vi "Initialize (Test).vi"() -> ()   [LabVIEW 2025]
uses:
  <vilib>/Instr/_visa.llb/VISA Open Access Mode.ctl
  <instrlib>/SMS LabVIEW Drivers/Labview Drivers/Cryogenic Ltd SMSXXX.lvlib
  <vilib>/regexp/Match Regular Expression.xnode
panel:
  in  "EOT Character (auto)":string="auto"
  in  "Serial Configuration":T1={"Baud Rate"=9600, "Parity"=0, "Data Bits"=8, "Stop Bits"=10, "Flow Control"=0} {"Flow Control" items=["None", "XON/XOFF", "RTS/CTS", "XON/XOFF & RTS/CTS", "DTR/DSR", "XON/XOFF & DTR/DSR"]; "Stop Bits" items=["1.0"=10, "1.5"=15, "2.0"=20]; "Data Bits" items=["7"=7, "8"=8]; "Parity" items=["None", "Odd", "Even", "Mark", "Space"]; "Baud Rate" items=["300"=300, "600"=600, "1200"=1200, "2400"=2400, "4800"=4800, "9600"=9600, "19200"=19200]}
  out "error out":errorcluster
  out "VISA Resource Name Out":refnum<visa-resource-name>
  in  "ID Query (True)":bool=TRUE
  in  "error in":errorcluster
  in  "APS VISA  IN":refnum<visa-resource-name>
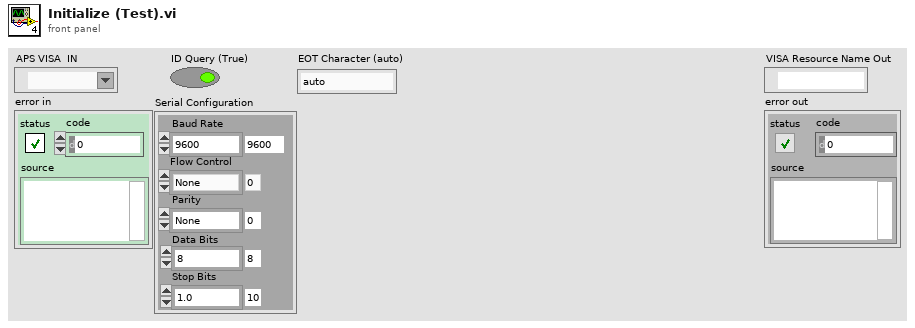
[diagram p1: front panel]
types:
  T1 = cluster{"Baud Rate":u32, "Parity":u16, "Data Bits":u16, "Stop Bits":u16, "Flow Control":u16}
  T2 = typedef "VISA Open Access Mode.ctl" = u32
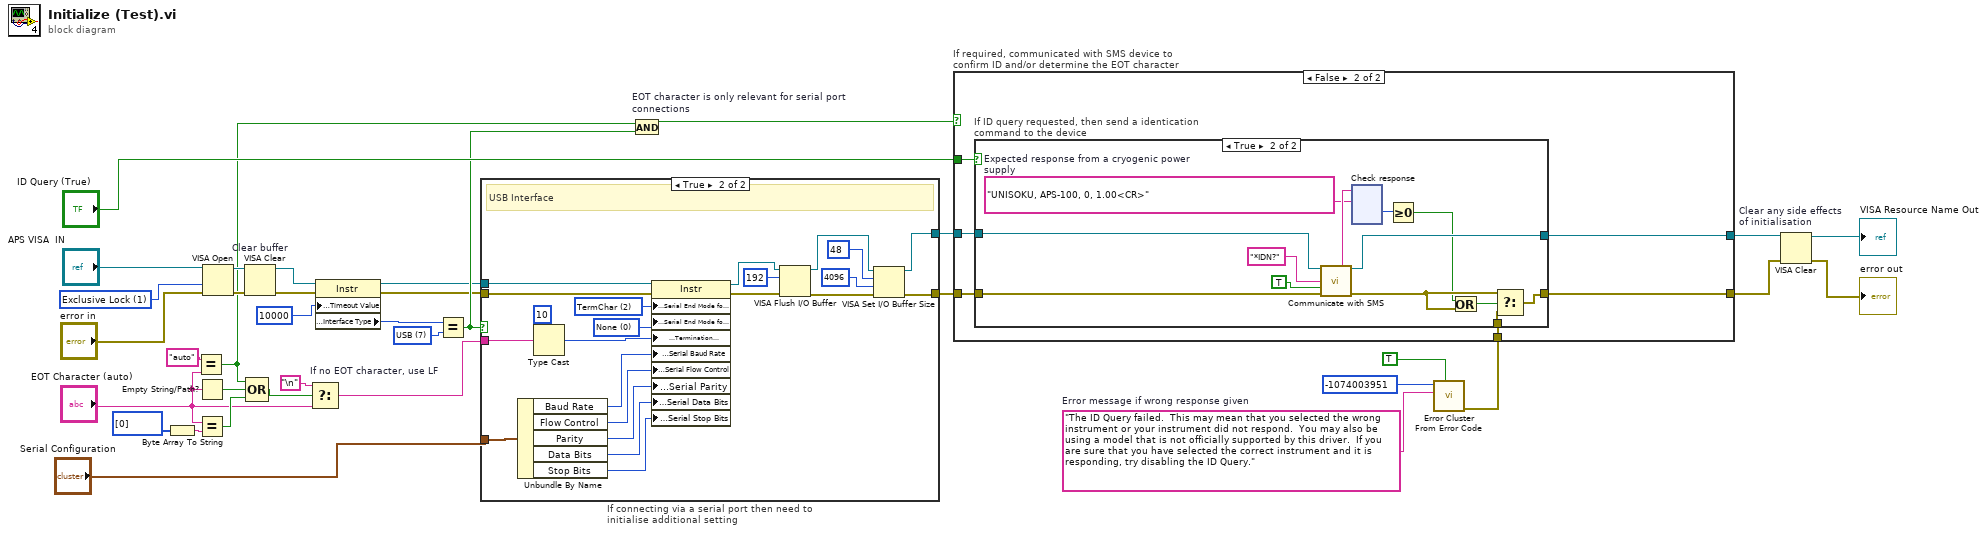
[diagram p0: block diagram]
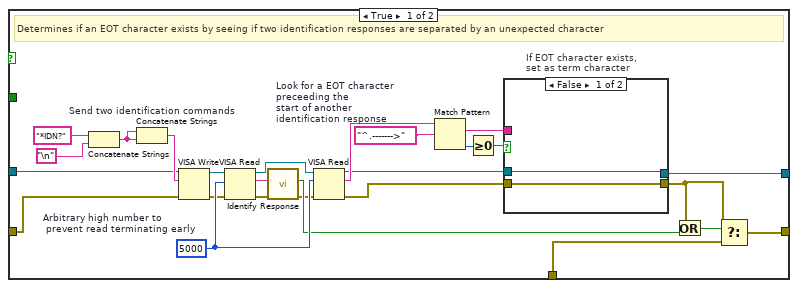
[diagram p2: hidden frame]
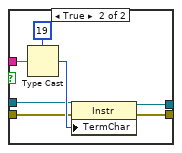
[diagram p3: hidden frame]
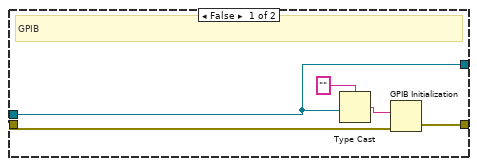
[diagram p5: hidden frame]
diagram:
  w23 = "The ID Query failed.  This may mean that you selected the wrong instrument or your instrument did not respond.  You may also be using a model that is not officially supported by this driver.  If you are sure that you have selected the correct instrument and it is responding, try disabling the ID Query."  # Error message if wrong response given
  w27 = T2 1 items=["VISA Defaults"=0, "Exclusive Lock"=1, "Load Configured Settings"=4] ("Access Mode")
  w33 = u16 7 items=["GPIB"=1, "VXI"=2, "GPIB-VXI"=3, "Serial"=4, "PXI"=5, "TCPIP"=6, "USB"=7] ("Interface Information:Interface Type")
  n1 = Byte Array To String(unsigned byte array=u8[] [0]) -> (string=w15:string)
  n2 = Equal?(x="auto", y="EOT Character (auto)") -> (x = y?=w4:bool)
  n3 = Empty String/Path?(string/path="EOT Character (auto)") -> (empty?=w20:bool)
  n4 = Equal?(x="EOT Character (auto)", y=w15) -> (x = y?=w14:bool)
  n5 = VISA Open(access mode=w27, error in (no error)="error in", VISA resource name="APS VISA  IN") -> (VISA resource name=w11:refnum<visa-resource-name>, error out=w10:errorcluster)  [unwired: 2 in]
  n6 = VISA Clear "Clear buffer"(VISA resource name=w11, error in (no error)=w10) -> (VISA resource name out=w34:refnum<visa-resource-name>, error out=w35:errorcluster)
  n7 = Compound Arithmetic op=OR(w4, w20, w14) -> (w19:bool)
  n8 = Select "If no EOT character, use LF"(t="\n", s=w19, f="EOT Character (auto)") -> (s? t:f=w17:string)
  n9 = property class="Instr"(reference=w34, error in=w35, "General Settings:Timeout Value"=u32 10000) -> (reference out=w1:refnum<visa-resource-name>, error out=w2:errorcluster, "Interface Information:Interface Type"=w36:u16)
  n10 = Equal?(x=w36, y=w33) -> (x = y?=w3:bool)
  n11 = case "If connecting via a serial port then need to initialise additional setting" shown="True" w3 {
    tunnel: [w40 w60] -> w28
    tunnel: w1 -> [w40 w62]
    tunnel: w2 -> [w37 w63]
    tunnel: [w38 w47] -> w29
    tunnel: "Serial Configuration" -> [_ w45]
    tunnel: w17 -> [_ w42]
    frame False {
      # "GPIB"
      n12 = Type Cast(type="", x=w40) -> (*(type *) &x=w41:string)
      n13 = GPIB Initialization(4:w37, 6:w41) -> (0:w38:errorcluster)  [unwired: 1 in, 4 out]
    }
    frame True {
      w46 = u16 0 items=["None", "Last Bit", "TermChar", "Break"] ("Serial Settings:End Mode for Writes")
      w53 = u16 2 items=["None", "LastBit", "TermChar"] ("Serial Settings:Serial End Mode for Reads")
      # "USB Interface"
      n14 = Unbundle By Name(w45) -> ("Baud Rate"=w52:u32, "Flow Control"=w49:u16, "Parity"=w50:u16, "Data Bits"=w51:u16, "Stop Bits"=w48:u16)
      n15 = Type Cast(type=u8 10 ("Message Based Settings:Termination Character"), x=w42) -> (*(type *) &x=w43:u8)
      n16 = property class="Instr"(reference=w62, error in=w63, "Serial Settings:Serial End Mode for Reads"=w53, "Serial Settings:Serial End Mode for Writes"=w46, "Message Based Settings:Termination Character"=w43, "Serial Settings:Serial Baud Rate"=w52, "Serial Settings:Serial Flow Control"=w49, "Serial Settings:Serial Parity"=w50, "Serial Settings:Serial Data Bits"=w51, "Serial Settings:Serial Stop Bits"=w48) -> (reference out=w57:refnum<visa-resource-name>, error out=w59:errorcluster)
      n17 = VISA Flush I/O Buffer(VISA resource name=w57, mask (16)=u16 192, error in (no error)=w59) -> (VISA resource name out=w61:refnum<visa-resource-name>, error out=w58:errorcluster)
      n18 = VISA Set I/O Buffer Size(VISA resource name=w61, mask (16)=u16 48, size (4096)=u32 4096 ("size (0)"), error in (no error)=w58) -> (VISA resource name out=w60:refnum<visa-resource-name>, error out=w47:errorcluster)
    }
  }
  n19 = And "EOT character is only relevant for serial port connections"(x=w4, y=w3) -> (x .and. y?=w5:bool)
  n20 = call <vilib>:"Error Cluster From Error Code.vi"("show call chain? (False)"=TRUE, "error message (\"\")"=w23, "error code (0)"=-1074003951 ("Code")) -> ("error out"=w22:errorcluster)  [unwired: 6 in]
  n21 = case "If required, communicated with SMS device to confirm ID and/or determine the EOT character" shown="False" w5 {
    tunnel: "ID Query (True)" -> [_ w104]
    tunnel: [w79 w103] -> w7
    tunnel: [w67 w102] -> w9
    tunnel: w29 -> [w83 w101]
    tunnel: w28 -> [w82 w100]
    tunnel: w22 -> [w78 w99]
    frame True {
      w85 = u32 5000  # Arbitrary high number to  prevent read terminating early
      # "Determines if an EOT character exists by seeing if two identification responses are separated by an unexpected character"
      n22 = Concatenate Strings("*IDN?", "\n") -> (w87:string)
      n23 = Concatenate Strings "Send two identification commands"(w87, w87) -> (w86:string)
      n24 = VISA Write(VISA resource name=w82, write buffer=w86, error in (no error)=w83) -> (VISA resource name out=w84:refnum<visa-resource-name>, error out=w72:errorcluster)  [unwired: 1 out]
      n25 = VISA Read(VISA resource name=w84, byte count=w85, error in (no error)=w72) -> (VISA resource name out=w68:refnum<visa-resource-name>, read buffer=w69:string, error out=w70:errorcluster)  [unwired: 1 out]
      n26 = call "Identify Response.vi"("error in"=w70, "Input String"=w69) -> ("error out"=w65:errorcluster, "Is SMS Response"=w66:bool)  [unwired: 8 in]
      n27 = VISA Read(VISA resource name=w68, byte count=w85, error in (no error)=w65) -> (VISA resource name out=w75:refnum<visa-resource-name>, read buffer=w81:string, error out=w74:errorcluster)  [unwired: 1 out]
      n28 = Match Pattern "Look for a EOT character preceeding the \nstart of another identification response"(string=w81, regular expression="^.------->") -> (match substring=w73:string, offset past match=w64:i32)  [unwired: 1 in, 2 out]
      n29 = Greater Or Equal To 0?(x=w64) -> (x >= 0?=w71:bool)
      n30 = case "If EOT character exists,\nset as term character" shown="False" w71 {
        tunnel: [w90 w98] -> w76
        tunnel: [w91 w97] -> w67
        tunnel: w75 -> [w91 w94]
        tunnel: w74 -> [w90 w95]
        tunnel: w73 -> [_ w93]
        frame False {
        }
        frame True {
          n31 = Type Cast(type=u8 19 ("Message Based Settings:Termination Character"), x=w93) -> (*(type *) &x=w96:u8)
          n32 = property class="Instr"(reference=w94, error in=w95, "TermChar"=w96) -> (reference out=w97:refnum<visa-resource-name>, error out=w98:errorcluster)
        }
      }
      n33 = Or(x=w76, y=w66) -> (x .or. y?=w80:bool)
      n34 = Select(t=w76, s=w80, f=w78) -> (s? t:f=w79:errorcluster)
    }
    frame False {
      n35 = case "If ID query requested, then send a identication command to the device" shown="True" w104 {
        tunnel: w100 -> [w106 w119]
        tunnel: w101 -> [w105 w118]
        tunnel: [w105 w107] -> w103
        tunnel: [w106 w112] -> w102
        tunnel: w99 -> [_ w108]
        frame False {
        }
        frame True {
          w113 = "UNISOKU, APS-100, 0, 1.00<CR>"  # Expected response from a cryogenic power supply
          n36 = call <instrlib>:"Communicate with SMS.vi"("VISA Resource Name In"=w119, "Query"="*IDN?", "Expected Answer? (F)"=TRUE ("Expected Answer?"), "error in (no error)"=w118) -> ("Answer"=w114:string, "VISA Resource Name Out"=w112:refnum<visa-resource-name>, "error out"=w110:errorcluster)  [unwired: 8 in, 1 out]
          n37 = xnode "Check response"("input string"=w114, "regular expression"=w113) -> ("offset past match"=w115:i32)  [unwired: 4 in, 4 out]
          n38 = Greater Or Equal To 0?(x=w115) -> (x >= 0?=w109:bool)
          n39 = Or(x=w109, y=w110) -> (x .or. y?=w111:bool)
          n40 = Select(t=w110, s=w111, f=w108) -> (s? t:f=w107:errorcluster)
        }
      }
    }
  }
  n41 = VISA Clear "Clear any side effects \nof initialisation"(VISA resource name=w9, error in (no error)=w7) -> (VISA resource name out=→"VISA Resource Name Out":refnum<visa-resource-name>, error out=→"error out":errorcluster)
